vi "Reply Dispatch Loop.vi"(8 "error in (no error)":errorcluster, 11 "TCPMessaging in":refnum<class "TCPMessaging.lvclass">) -> (0 "error out":errorcluster)   [LabVIEW 2020, in "Vecto.lvlib" / "TCPMessaging.lvclass"]
uses:
  TCPMessaging.lvclass
  Reply Dispatch Loop Data.ctl
  Request Registration.ctl
  <vilib>/IlluminatedG/IG Promises/Promises/Promise/Promise.lvclass
  TCPMessaging.lvclass/TCPMessaging.ctl
  <vilib>/IlluminatedG/IG Promises/Promises/Value/Value.lvclass
  106ad472-1f31-4d7c-a09c-120c0a133575.vi
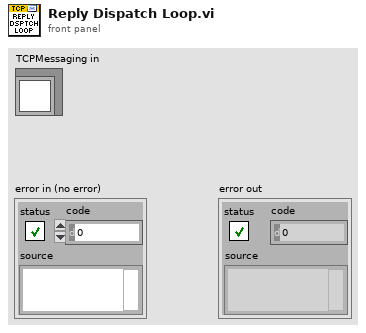
[diagram p1: front panel]
types:
  T1 = typedef "Vecto.lvlib/TCPMessaging.lvclass/Reply Dispatch Loop Data.ctl" = cluster{"Requests":map{u32, T2}}
  T2 = typedef "Vecto.lvlib/TCPMessaging.lvclass/Request Registration.ctl" = cluster{"Sequence":u32, "Reply Promise":refnum<class "Promise.lvclass">, "Reply Deadline":dbl}
  T3 = typedef "TcpPayload.lvlib/Data.ctl" = cluster{"target_node":u32, "target_task":u32, "source_id":u32, "sequence":u32, "timestamp":u64, "type_id":u32, "payload":u8[]}
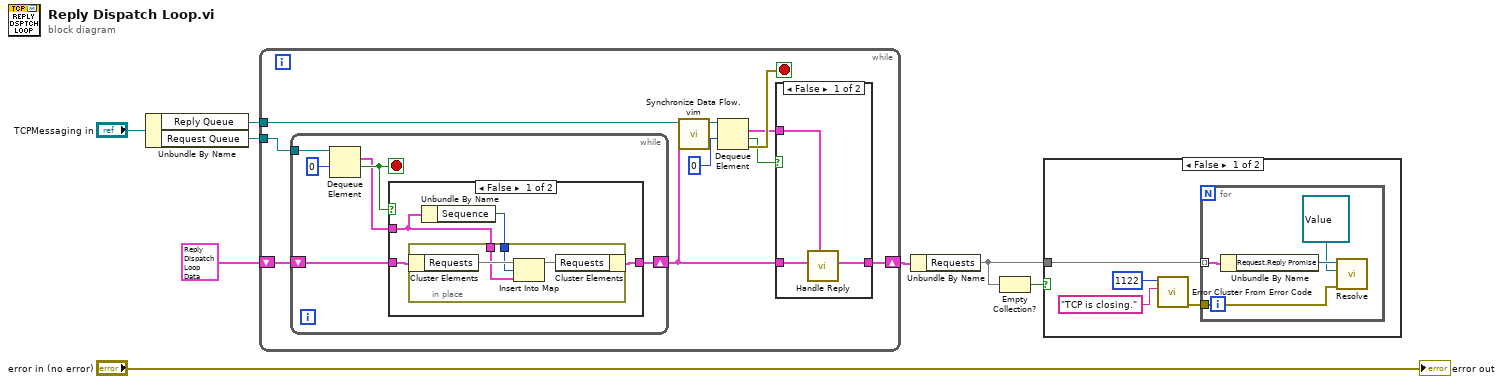
[diagram p0: block diagram]
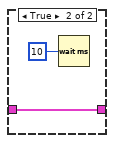
[diagram p3: hidden frame]
diagram:
  n1 = Unbundle By Name("TCPMessaging in") -> ("Reply Queue"=w4:refnum<queue>, "Request Queue"=w6:refnum<queue>)
  n2 = while {
    tunnel: w6 -> [w16]
    shift-right: [w9] -> w3
    shift-left: T1 {"Requests"={}} ("Reply Dispatch Loop Data") -> [w17]
    tunnel: w4 -> [w15]
    stop <- w18 stop-if-true
    n3 = while {
      shift-right: [w25] -> w10
      shift-left: w17 -> [w24]
      tunnel: w16 -> [w29]
      stop <- w27 stop-if-true
      n4 = Dequeue Element(queue=w29, timeout in ms (-1)=0) -> (element=w26:T2, timed out?=w27:bool)  [unwired: 1 in, 2 out]
      n5 = case shown="False" w27 {
        tunnel: w26 -> [w30 _]
        tunnel: [w32 w38] -> w25
        tunnel: w24 -> [w33 w38]
        frame False {
          n6 = Unbundle By Name(w30) -> ("Sequence"=w31:u32)
          n7 = in-place {
            in-place-border: w31 -> [w35]
            in-place-border: w30 -> [w34]
            n8 = in-place-cluster #1(w33) -> ("Requests"=w37:map{u32, T2})
            n9 = Insert Into Map(map in=w37, key=w35, value=w34) -> (map out=w36:map{u32, T2})  [unwired: 2 out]
            n10 = in-place-cluster #1("Requests"=w36) -> (w32:T1)
          }
        }
        frame True {
        }
      }
    }
    n11 = call "Synchronize Data Flow.vim"("input 4"=w10, "input 1"=w15) -> ("output 1"=w14:refnum<queue>)  [unwired: 2 in, 3 out]
    n12 = Dequeue Element(queue=w14, timeout in ms (-1)=0) -> (element=w11:T3, timed out?=w12:bool, error out=w18:errorcluster)  [unwired: 1 in, 1 out]
    n13 = case shown="False" w12 {
      tunnel: w11 -> [w20 _]
      tunnel: w10 -> [w21 w23]
      tunnel: [w19 w23] -> w9
      frame False {
        n14 = call "Handle Reply.vi"("TcpPayload"=w20, "Reply Dispatch Loop Data in"=w21) -> ("Reply Dispatch Loop Data"=w19:T1)  [unwired: 9 in]
      }
      frame True {
        n15 = Wait (ms)(milliseconds to wait=u32 10) -> ()  [unwired: 1 out]
      }
    }
  }
  n16 = Unbundle By Name(w3) -> ("Requests"=w2:map{u32, T2})
  n17 = Empty Collection?(1:w2) -> (0:w1:bool)
  n18 = case shown="False" w1 {
    tunnel: w2 -> [w42 _]
    frame False {
      n19 = call <vilib>:"Error Cluster From Error Code.vi"("error message (\"\")"="TCP is closing." ("error message (\"\")"), "error code (0)"=1122) -> ("error out"=w39:errorcluster)  [unwired: 7 in]
      n20 = for {
        tunnel: w42 -> [w46] mode=indexing
        tunnel: w39 -> [w44]
        n21 = Unbundle By Name(w46) -> ("Request.Reply Promise"=w45:refnum<class "Promise.lvclass">)
        n22 = call <vilib>:"Resolve.vi"("error in (no error)"=w44, "Result"=refnum<class "Value.lvclass"> refnum, "Promise in"=w45) -> ()  [unwired: 7 in, 2 out]
      }
    }
    frame True {
    }
  }
  "error out" <- "error in (no error)"
